vi "Get Target Info.vi"(7 "force property refresh (T)":bool=TRUE, 8 "error in (no error)":errorcluster, 11 "target":string) -> (0 "error out":errorcluster, 3 "target info":T1 {"IP Mode" items=["Static"=1, "DHCP/Link-Local"=2, "Link-Local Only"=4, "DHCP Only"=8]})   [LabVIEW 2013]
uses:
  types/MAX Sys Cfg Target Information.ctl
  <vilib>/nisyscfg/Initialize (String).vi
  <vilib>/nisyscfg/Close (System).vi
  <vilib>/nisyscfg/nisyscfg.lvlib
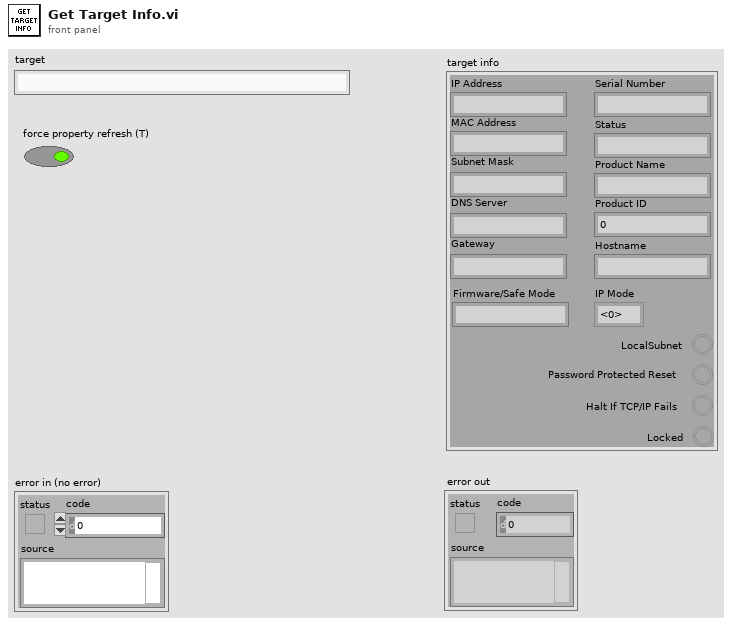
[diagram p1: front panel]
types:
  T1 = typedef "MAX Sys Cfg Target Information.ctl" = cluster{"MAC Address":string, "IP Address":string, "Status":string, "Product Name":string, "Hostname":string, "Firmware/Safe Mode":string, "Subnet Mask":string, "Gateway":string, "DNS Server":string, "Serial Number":string, "Product ID":u32, "Locked ":bool, "LocalSubnet":bool, "Halt If TCP/IP Fails":bool, "Password Protected Reset":bool, "IP Mode":i32}
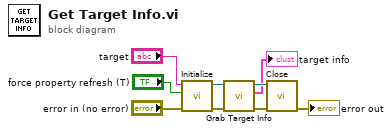
[diagram p0: block diagram]
diagram:
  n1 = call-poly <vilib>:"Initialize.vi"("error in (no error)"="error in (no error)", "force property refresh (T)"="force property refresh (T)", "target (localhost)"="target") -> ("error out"=w7:errorcluster, "session out"=w8:refnum<k21>)  [unwired: 6 in, 1 out]
  n2 = call "Grab Target Info.vi"("error in (no error)"=w7, "Refnum in"=w8) -> ("error out"=w6:errorcluster, "Network Module Information"=→"target info":T1, "Refnum out"=w5:refnum<k21>)  [unwired: 7 in]
  n3 = call-poly <vilib>:"Close.vi"("error in (no error)"=w6, "session in"=w5) -> ("error out"=→"error out":errorcluster)  [unwired: 9 in]
